vi "E-Fuse Readback.vi"(7 "write buffer":string, 8 "error in (no error)":errorcluster, 9 "delay before read (ms)":u32=100, 10 "Init":bool, 11 "VISA resource name":refnum<visa-resource-name>="COM1") -> (0 "error out":errorcluster, 2 "EFuse Read Back":string, 3 "VISA resource name out":refnum<visa-resource-name>)   [LabVIEW 2017]
panel:
  out "read buffer":string
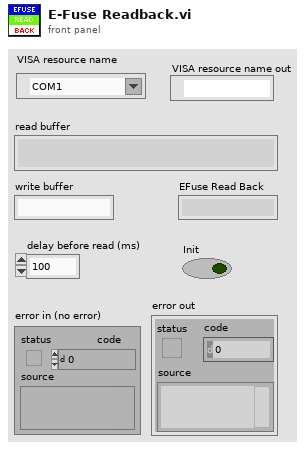
[diagram p1: front panel]
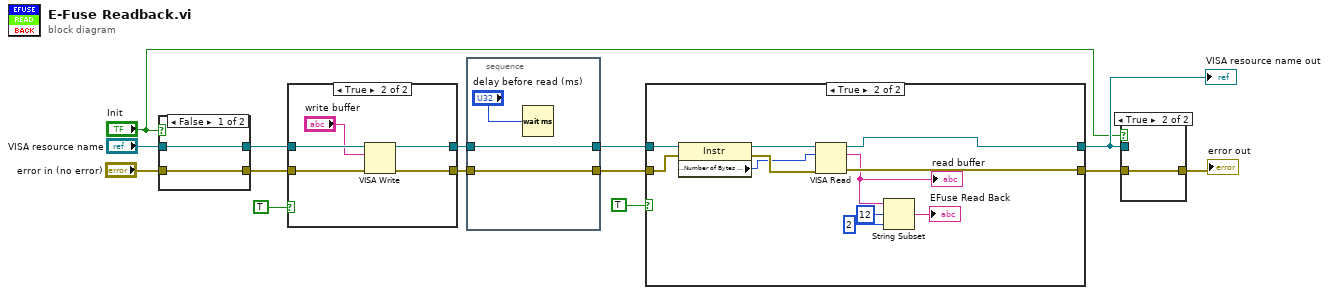
[diagram p0: block diagram]
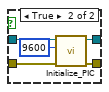
[diagram p3: hidden frame]
diagram:
  n1 = case shown="False" "Init" {
    tunnel: [w15 w21] -> w8
    tunnel: [w16 w20] -> w7
    tunnel: "VISA resource name" -> [w16 w19]
    tunnel: "error in (no error)" -> [w15 w18]
    frame False {
    }
    frame True {
      n2 = call "Initialize_PIC.vi"("error in (no error)"=w18, "baud rate"=u32 9600, "Select Com Port"=w19) -> ("error out"=w21:errorcluster, "VISA resource name out"=w20:refnum<visa-resource-name>)  [unwired: 7 in]
    }
  }
  n3 = case shown="True" TRUE {
    tunnel: [w23 w28] -> w14
    tunnel: w7 -> [w22 w27]
    tunnel: w8 -> [w23 w26]
    tunnel: [w22 w25] -> w12
    frame False {
    }
    frame True {
      n4 = VISA Write(VISA resource name=w27, write buffer="write buffer", error in (no error)=w26) -> (VISA resource name out=w25:refnum<visa-resource-name>, error out=w28:errorcluster)  [unwired: 1 out]
    }
  }
  n5 = stacked-sequence {
    tunnel: w14 -> [w31]
    tunnel: [w31] -> w13
    tunnel: w12 -> [w30]
    tunnel: [w30] -> w11
    frame #0 {
      n6 = Wait (ms)(milliseconds to wait="delay before read (ms)") -> ()  [unwired: 1 out]
    }
  }
  n7 = case shown="True" TRUE {
    tunnel: w13 -> [w33 w42]
    tunnel: [w33 w35] -> w4
    tunnel: [w32 w36] -> w2
    tunnel: w11 -> [w32 w44]
    frame False {
    }
    frame True {
      n8 = property class="Instr"(reference=w44, error in=w42) -> (reference out=w43:refnum<visa-resource-name>, error out=w41:errorcluster, "Serial Settings:Number of Bytes at Serial Port"=w39:u32)
      n9 = VISA Read(VISA resource name=w43, byte count=w39, error in (no error)=w41) -> (VISA resource name out=w36:refnum<visa-resource-name>, read buffer=w34:string, error out=w35:errorcluster)  [unwired: 1 out]
      "read buffer" <- w34
      n10 = String Subset(string=w34, offset (0)=12, length (rest)=2 ("length (rest)")) -> (substring=→"EFuse Read Back":string)
    }
  }
  "VISA resource name out" <- w2
  n11 = case shown="True" "Init" {
    tunnel: w4 -> [w45 w46]
    tunnel: [w45 w46] -> w3
    tunnel: w2 -> [_ _]
    frame False {
    }
    frame True {
    }
  }
  "error out" <- w3
